vi "WSVCAP SHL FPGA LL I2C Read Data.vi"(11 "error in (no error)":errorcluster, 12 "UUT Set (0-1) (Legacy)":u8, 13 "Socket Mask":u64 format="%012x") -> (4 "Long Word Out (1-Bit for Each Channel)":u64, 15 "error out":errorcluster)   [LabVIEW 2017]
uses:
  WSVCAP SHL FPGA LL I2C Debug Global.vi
  <vilib>/eio/EIONode/EIONode.xnode
  <vilib>/rvi/eio/common/nirviEmuTemplateMethod_errors.vi
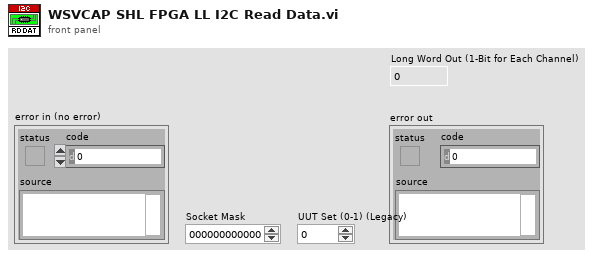
[diagram p1: front panel]
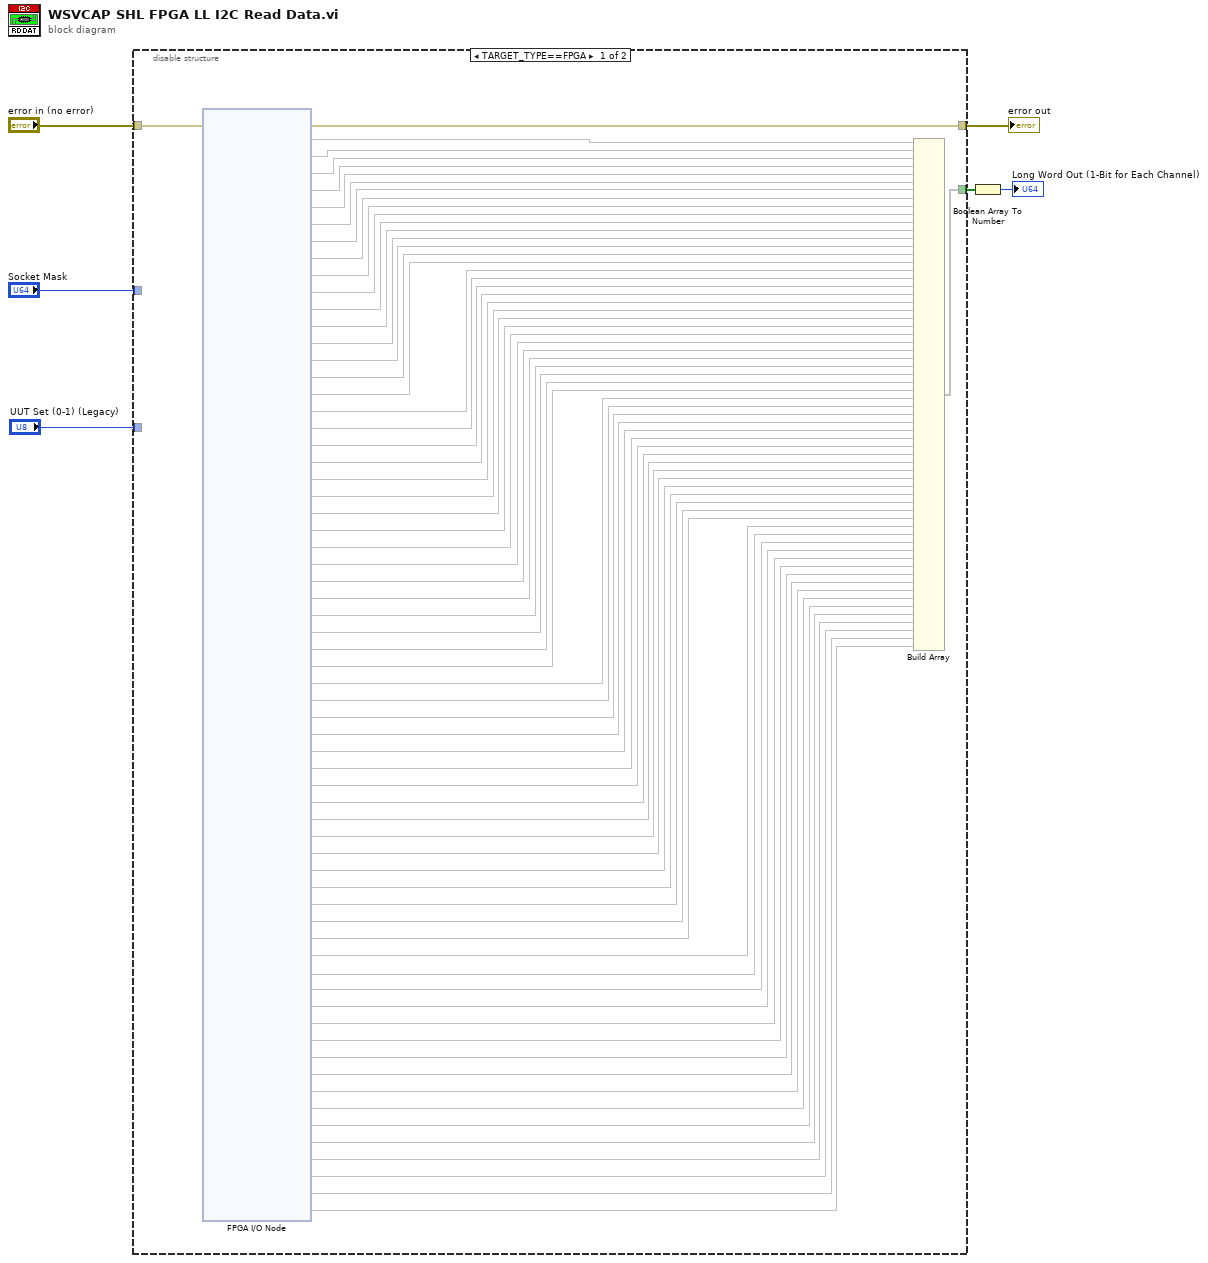
[diagram p0: block diagram]
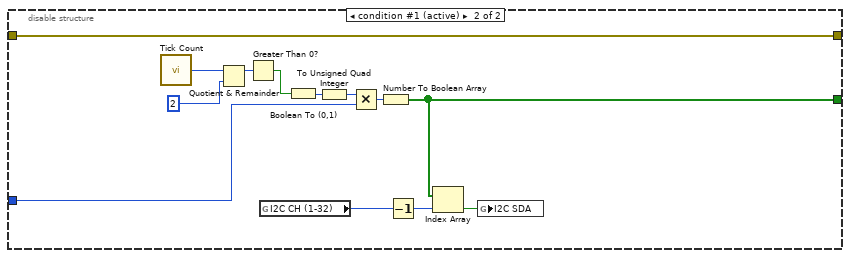
[diagram p2: hidden frame]
diagram:
  n1 = disable-structure shown="TARGET_TYPE==FPGA" {
    disable-tunnel: [w73 w83] -> w6
    disable-tunnel: "error in (no error)" -> [w72 w83]
    disable-tunnel: "Socket Mask" -> [_ w80]
    disable-tunnel: [w38 w74] -> w2
    disable-tunnel: "UUT Set (0-1) (Legacy)" -> [_ _]
    frame condition #0 {
      n2 = xnode "FPGA I/O Node"("error in"=w72) -> ("error out"=w73:errorcluster, "I2C_SDA_S1"=w71, "I2C_SDA_S2"=w70, "I2C_SDA_S3"=w69, "I2C_SDA_S4"=w68, "I2C_SDA_S5"=w67, "I2C_SDA_S6"=w66, "I2C_SDA_S7"=w65, "I2C_SDA_S8"=w64, "I2C_SDA_S9"=w63, "I2C_SDA_S10"=w62, "I2C_SDA_S11"=w61, "I2C_SDA_S12"=w60, "I2C_SDA_S13"=w59, "I2C_SDA_S14"=w58, "I2C_SDA_S15"=w57, "I2C_SDA_S16"=w37, "I2C_SDA_S17"=w36, "I2C_SDA_S18"=w56, "I2C_SDA_S19"=w55, "I2C_SDA_S20"=w54, "I2C_SDA_S21"=w53, "I2C_SDA_S22"=w52, "I2C_SDA_S23"=w51, "I2C_SDA_S24"=w50, "I2C_SDA_S25"=w49, "I2C_SDA_S26"=w48, "I2C_SDA_S27"=w47, "I2C_SDA_S28"=w46, "I2C_SDA_S29"=w45, "I2C_SDA_S30"=w44, "I2C_SDA_S31"=w43, "I2C_SDA_S32"=w42, "I2C_SDA_S33"=w41, "I2C_SDA_S34"=w40, "I2C_SDA_S35"=w39, "I2C_SDA_S36"=w35, "I2C_SDA_S37"=w34, "I2C_SDA_S38"=w33, "I2C_SDA_S39"=w32, "I2C_SDA_S40"=w31, "I2C_SDA_S41"=w30, "I2C_SDA_S42"=w29, "I2C_SDA_S43"=w28, "I2C_SDA_S44"=w27, "I2C_SDA_S45"=w26, "I2C_SDA_S46"=w25, "I2C_SDA_S47"=w24, "I2C_SDA_S48"=w23, "I2C_SDA_S49"=w22, "I2C_SDA_S50"=w21, "I2C_SDA_S51"=w20, "I2C_SDA_S52"=w19, "I2C_SDA_S53"=w18, "I2C_SDA_S54"=w17, "I2C_SDA_S55"=w16, "I2C_SDA_S56"=w15, "I2C_SDA_S57"=w14, "I2C_SDA_S58"=w13, "I2C_SDA_S59"=w12, "I2C_SDA_S60"=w11, "I2C_SDA_S61"=w10, "I2C_SDA_S62"=w9, "I2C_SDA_S63"=w8, "I2C_SDA_S64"=w7)  [unwired: 64 in, 64 out]
      n3 = Build Array(w71, w70, w69, w68, w67, w66, w65, w64, w63, w62, w61, w60, w59, w58, w57, w37, w36, w56, w55, w54, w53, w52, w51, w50, w49, w48, w47, w46, w45, w44, w43, w42, w41, w40, w39, w35, w34, w33, w32, w31, w30, w29, w28, w27, w26, w25, w24, w23, w22, w21, w20, w19, w18, w17, w16, w15, w14, w13, w12, w11, w10, w9, w8, w7) -> (w38:void[])
    }
    frame condition #1 (active) {
      n4 = call "Tick Count"() -> ("Tick Count(Ticks)"=w86:u32)
      n5 = Quotient & Remainder(x=w86, y=u32 2) -> (x-y*floor(x/y)=w85:u32)  [unwired: 1 out]
      n6 = Greater Than 0?(x=w85) -> (x > 0?=w82:bool)
      n7 = global read "WSVCAP SHL FPGA LL I2C Debug Global.vi" "I2C CH (1-32)"() -> (w79:i32)
      n8 = Boolean To (0,1)(Boolean=w82) -> (0, 1=w81:i16)
      n9 = To Unsigned Quad Integer(1:w81) -> (0:w78:u64)
      n10 = Multiply(x=w78, y=w80) -> (x*y=w77:u64)
      n11 = Number To Boolean Array(number=w77) -> (Boolean array=w74:bool[])
      n12 = Decrement(x=w79) -> (x-1=w75:i32)
      n13 = Index Array(array=w74, index=w75) -> (element=w76:bool)
      n14 = global write "WSVCAP SHL FPGA LL I2C Debug Global.vi" "I2C SDA"(w76) -> ()
    }
  }
  "error out" <- w6
  n15 = Boolean Array To Number(Boolean array=w2) -> (number=→"Long Word Out (1-Bit for Each Channel)":u64)
